vi "loadTestsFromTestTag.vi"(7 "testSuiteStatusChangedRef":refnum<user-event>, 8 "error in (no error)":errorcluster, 10 "Tests":refnum<class>[](array[class]), 11 "TestLoader in":refnum<class "TestLoader.lvclass">) -> (0 "error out":errorcluster, 2 "TestSuite":refnum<class "TestSuite.lvclass">, 3 "TestLoader out":refnum<class "TestLoader.lvclass">)   [LabVIEW 2013, in "TestLoader.lvclass"]
uses:
  TestLoader.lvclass
  TestSuite/TestSuite.lvclass
  TestSuite/suiteStatusChanged--Cluster.ctl
  TestSuite/suiteStatus--enum.ctl
panel:
  # "JKI VI Tester for LabVIEW\nhttp://jkisoft.com/vi-tester\nCopyright (C) 2007-2009, JKI <info@jkisoft.com>\nALL RIGHTS RESERVED"
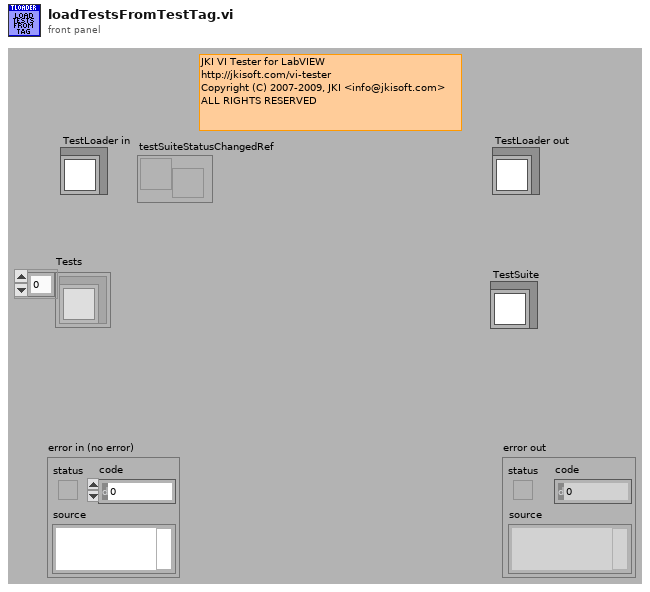
[diagram p1: front panel]
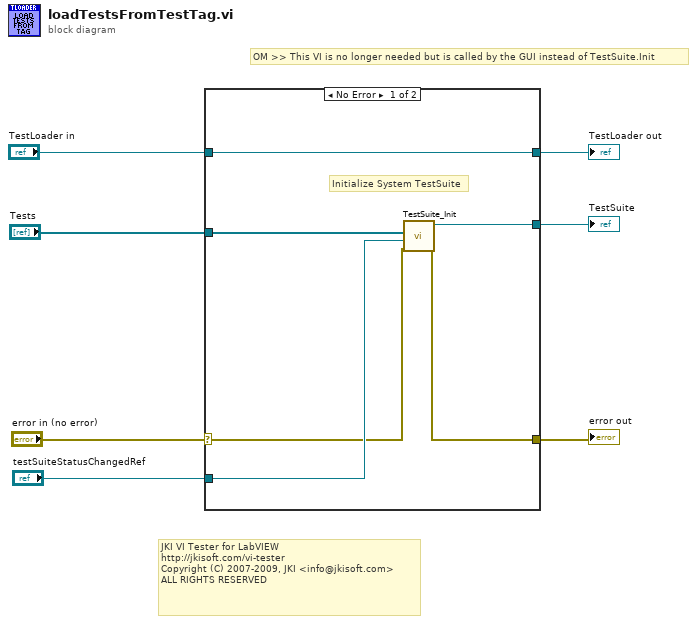
[diagram p0: block diagram]
diagram:
  # "OM >> This VI is no longer needed but is called by the GUI instead of TestSuite.Init"
  # "JKI VI Tester for LabVIEW\nhttp://jkisoft.com/vi-tester\nCopyright (C) 2007-2009, JKI <info@jkisoft.com>\nALL RIGHTS RESERVED"
  n1 = case shown="No Error" "error in (no error)" {
    selector: "error in (no error)" -> [w9 w15]
    tunnel: [w11 w15] -> w6
    tunnel: [w13 w14] -> w4
    tunnel: "TestLoader in" -> [w13 w14]
    tunnel: "Tests" -> [w8 _]
    tunnel: [w12 _] -> w2
    tunnel: "testSuiteStatusChangedRef" -> [w10 _]
    frame No Error {
      # "Initialize System TestSuite"
      n2 = call "TestSuite_Init.vi"("error in (no error)"=w9, "testSuiteStatusChanged EventRef"=w10, "tests (none)"=w8) -> ("error out"=w11:errorcluster, "TestSuite out"=w12:refnum<class "TestSuite.lvclass">)  [unwired: 7 in]
    }
    frame Error {
    }
  }
  "error out" <- w6
  "TestLoader out" <- w4
  "TestSuite" <- w2
